vi "PI-TF.vi"(4 "reset-val":sgl format="%#_13g", 5 "u(k-1)":sgl format="%#_13g", 6 "reset":bool, 8 "Ki":sgl, 9 "setpoint":sgl, 11 "y(k)":sgl format="%#_13g") -> (1 "u(k)":sgl)   [LabVIEW 2015]
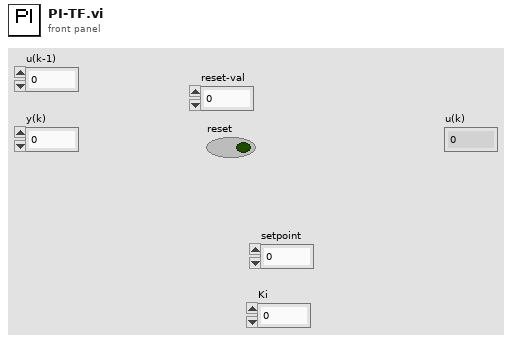
[diagram p1: front panel]
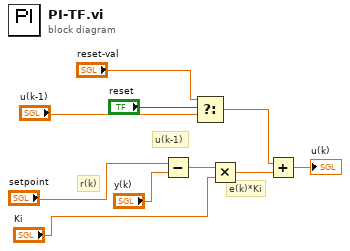
[diagram p0: block diagram]
diagram:
  # "e(k)*Ki"
  # "u(k-1)"
  # "r(k)"
  n1 = Subtract(x="setpoint", y="y(k)") -> (x-y=w10:sgl)
  n2 = Select(t="reset-val", s="reset", f="u(k-1)") -> (s? t:f=w5:sgl)
  n3 = Multiply(x=w10, y="Ki") -> (x*y=w9:sgl)
  n4 = Add(x=w5, y=w9) -> (x+y=→"u(k)":sgl)
